vi "ROI entry screen-main buttons management.vi"(6 "Imaging button boolean text":string=". . .", 7 "Acquisition button boolean text":string=". . .", 8 "Imaging button disabled?":T1(ring), 9 "Acquisition button disabled?":T1(ring), 10 "Done button disabled?":T1(ring)) -> ()   [LabVIEW 2017]
uses:
  Typedefs/Read Write Enum.ctl
  Globals/gl_ROI Entry UI globals.vi
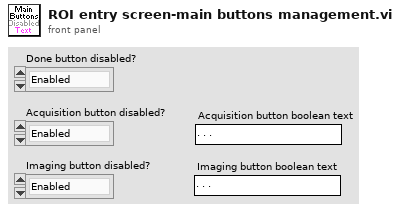
[diagram p1: front panel]
types:
  T1 = enum8{"Enabled", "Disabled", "Disabled and Grayed Out"}
  T2 = typedef "Read Write Enum.ctl" = enum16{"Read", "Write"}
  T3 = typedef "ROI entry screen ctrl refs cluster.ctl" = cluster{"Done button":refnum<vi>, "Imaging button":refnum<vi>, "Acquisition button":refnum<vi>, "POI dwell time (us)":refnum<vi>, "Scan dwell time per pixel (us)":refnum<vi>, "# of planes":refnum<vi>, "Zoom Ctrl":refnum<vi>, "Equal size":refnum<vi>, "Channel":refnum<vi>, "Image Display":refnum<vi>, "Z-Plane Selector":refnum<vi>, "Number of lines left":refnum<vi>, "Z-stack folder path":refnum<vi>, "POI Density":refnum<vi>, "Arb Plane Entry":refnum<vi>, "Whole plane":refnum<vi>, "Clear Last":refnum<vi>, "Clear All":refnum<vi>, "Trial Length (sec)":refnum<vi>, "Palette Type":refnum<vi>, "Intensity slider":refnum<vi>, "# POI":refnum<vi>, "Max Z Proj":refnum<vi>, "Zplane ind":refnum<vi>, "Wavelength (nm)":refnum<vi>, "Number of Trials":refnum<vi>, "Funct stim.trig.enable":refnum<vi>, "Funct stim.trig.delay (s)":refnum<vi>, "Line Mode":refnum<vi>, "Step size (µm)":refnum<vi>, "ROI move mode":refnum<vi>, "Cool-down time (s)":refnum<vi>, "Enable cool-down time":refnum<vi>, "Motor Z ind. (um)":refnum<vi>, "AOL Z ind. (um)":refnum<vi>, "Load Reference Image":refnum<vi>}
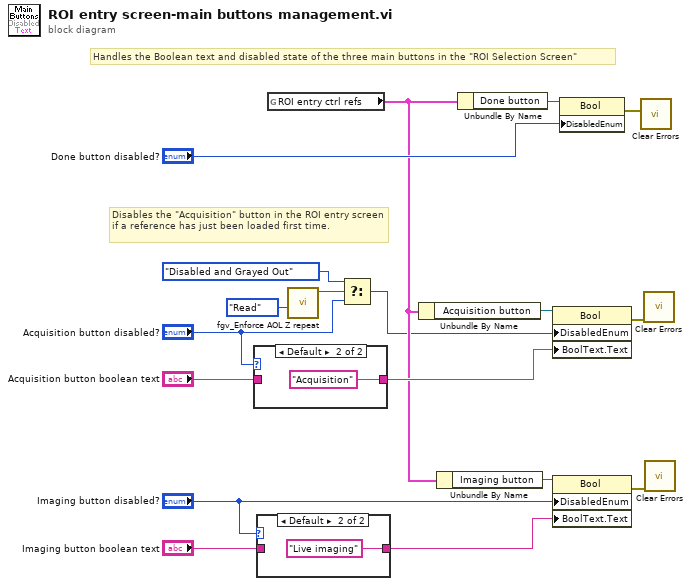
[diagram p0: block diagram]
diagram:
  # "Disables the \"Acquisition\" button in the ROI entry screen if a reference has just been loaded first time."
  # "Handles the Boolean text and disabled state of the three main buttons in the \"ROI Selection Screen\""
  n1 = case shown="Default" "Acquisition button disabled?" {
    tunnel: [w19 "Acquisition" ("Boolean Text.Text")] -> w10
    tunnel: "Acquisition button boolean text" -> [w19 _]
    frame "Enabled" {
    }
    frame Default {
    }
  }
  n2 = case shown="Default" "Imaging button disabled?" {
    tunnel: [w21 "Live imaging" ("Boolean Text.Text")] -> w15
    tunnel: "Imaging button boolean text" -> [w21 _]
    frame "Enabled" {
    }
    frame Default {
    }
  }
  n3 = global read "gl_ROI Entry UI globals.vi" "ROI entry ctrl refs"() -> (w9:T3)
  n4 = call "fgv_Enforce AOL Z repeat.vi"("Function"=Read_Write_Enum."Read") -> ("Enforce AOL Z repeat?"=w4:bool)  [unwired: 9 in, 1 out]
  n5 = Select(t=T1."Disabled and Grayed Out" ("Disabled"), s=w4, f="Acquisition button disabled?") -> (s? t:f=w1:T1)
  n6 = Unbundle By Name(w9) -> ("Acquisition button"=w13:refnum<vi>)
  n7 = Unbundle By Name(w9) -> ("Imaging button"=w14:refnum<vi>)
  n8 = Unbundle By Name(w9) -> ("Done button"=w18:refnum<vi>)
  n9 = property on="Property Node" class="Bool"(reference=w13, "DisabledEnum"=w1, "BoolText.Text"=w10) -> (error out=w6:errorcluster)  [unwired: 1 in, 1 out]
  n10 = property on="Property Node" class="Bool"(reference=w14, "DisabledEnum"="Imaging button disabled?", "BoolText.Text"=w15) -> (error out=w7:errorcluster)  [unwired: 1 in, 1 out]
  n11 = property on="Property Node" class="Bool"(reference=w18, "DisabledEnum"="Done button disabled?") -> (error out=w8:errorcluster)  [unwired: 1 in, 1 out]
  n12 = call <vilib>:"Clear Errors.vi"("error in (no error)"=w8) -> ()  [unwired: 5 in, 2 out]
  n13 = call <vilib>:"Clear Errors.vi"("error in (no error)"=w6) -> ()  [unwired: 5 in, 2 out]
  n14 = call <vilib>:"Clear Errors.vi"("error in (no error)"=w7) -> ()  [unwired: 5 in, 2 out]
